vi "Read diagonalLength.vi"(8 "error in (no error)":errorcluster, 11 "Field in":refnum<class "Field.lvclass">) -> (0 "error out":errorcluster, 2 "diagonalLength":dbl, 3 "Field out":refnum<class "Field.lvclass">)   [LabVIEW 2023, in "Field.lvclass"]
uses:
  Field.lvclass
  Field.lvclass/Field.ctl
  <vilib>/Analysis/_algsub.llb/Real Vector Norm.vi
  <vilib>/Analysis/NI_AALPro.lvlib
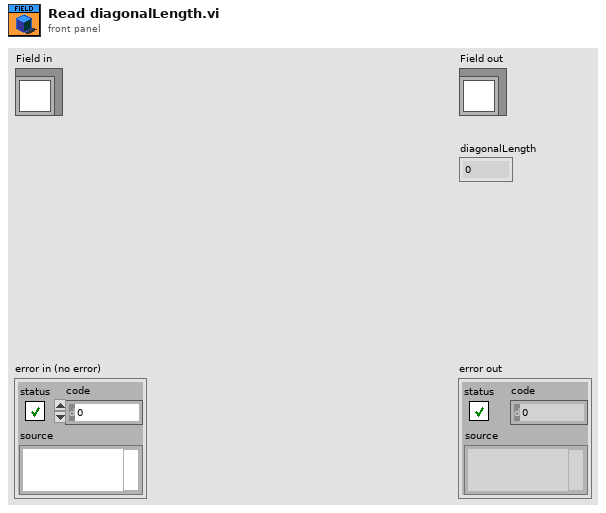
[diagram p1: front panel]
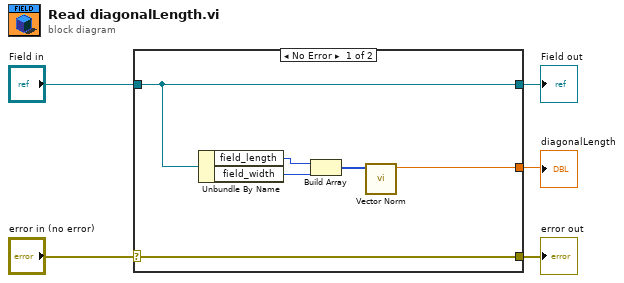
[diagram p0: block diagram]
diagram:
  n1 = case shown="No Error" "error in (no error)" {
    selector: "error in (no error)" -> [w11 w12]
    tunnel: [w11 w12] -> w4
    tunnel: [w8 w13] -> w2
    tunnel: "Field in" -> [w8 w13]
    tunnel: [w6 _] -> w1
    frame No Error {
      n2 = Unbundle By Name(w8) -> ("field_length"=w9:i32, "field_width"=w10:i32)
      n3 = Build Array(w9, w10) -> (w7:i32[])
      n4 = call-poly <vilib>:"Vector Norm.vi"("Input Vector"=w7) -> ("norm"=w6:dbl)  [unwired: 9 in, 1 out]
    }
    frame Error {
    }
  }
  "error out" <- w4
  "Field out" <- w2
  "diagonalLength" <- w1
